vi "Serial Interface.vi"(1 "UART Inputs":T2={"Tx Data"=[0, 0, 0, 0, 0, 0, 0, 0, 0, 0], "Transmit"=FALSE, "Receive"=FALSE, "Byte Mode"=TRUE, "Set Baud Rate"=FALSE, "Baud Rate"=0} {"Baud Rate" format="%02x"; "Tx Data" format="%02x"}) -> (0 "UART Outputs":T1 {"Rx Data" format="%02x"})   [LabVIEW 2016]
uses:
  <vilib>/rvi/eio/common/nirviEmuTemplateMethod_errors.vi
  <vilib>/eio/EIONode/EIONode.xnode
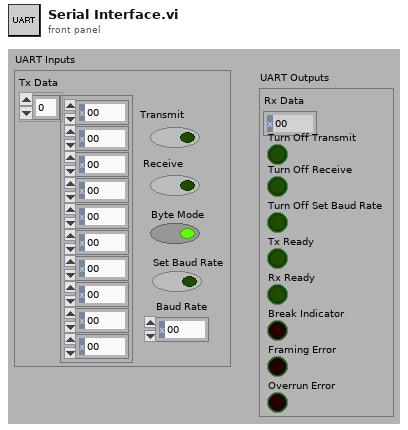
[diagram p1: front panel]
types:
  T1 = cluster{"Rx Data":u8, "Turn Off Transmit":bool, "Turn Off Receive":bool, "Turn Off Set Baud Rate":bool, "Tx Ready":bool, "Rx Ready":bool, "Break Indicator":bool, "Framing Error":bool, "Overrun Error":bool}
  T2 = cluster{"Tx Data":u8[], "Transmit":bool, "Receive":bool, "Byte Mode":bool, "Set Baud Rate":bool, "Baud Rate":u8}
  T3 = enum16{"Idle", "Assert Read", "Latch Data", "Done"}
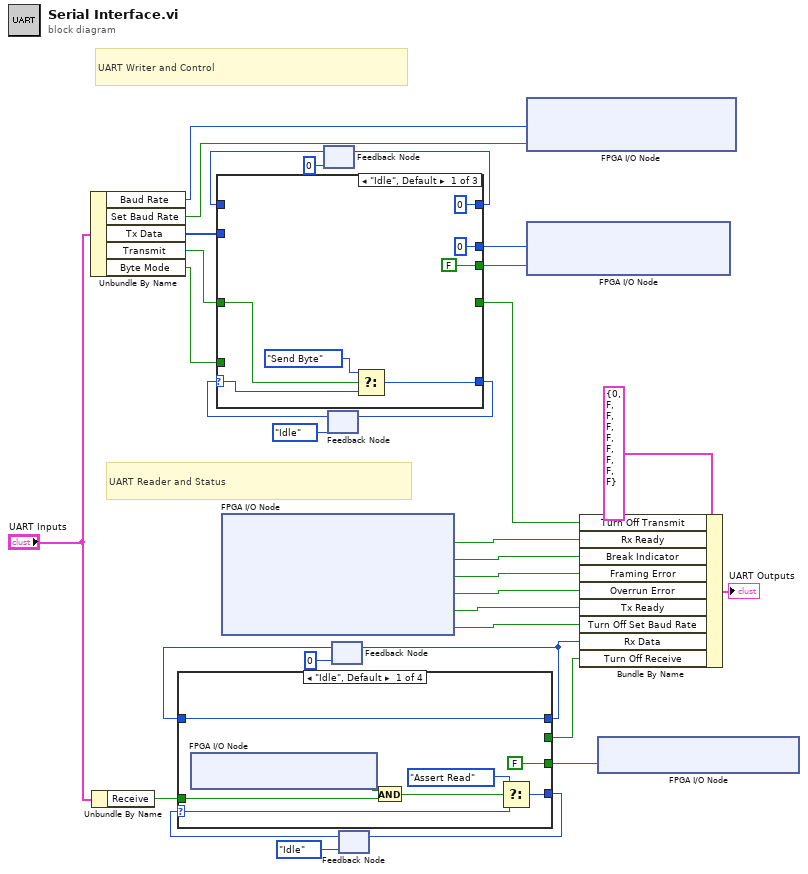
[diagram p0: block diagram]
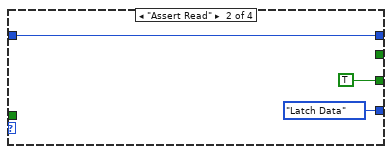
[diagram p2: hidden frame]
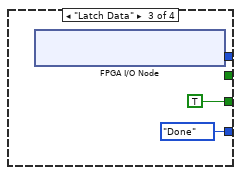
[diagram p3: hidden frame]
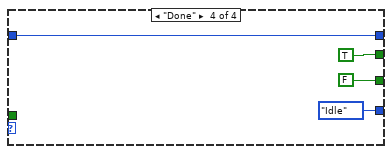
[diagram p4: hidden frame]
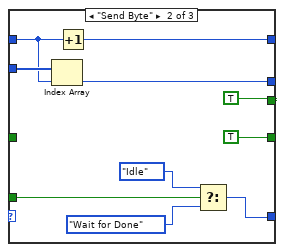
[diagram p5: hidden frame]
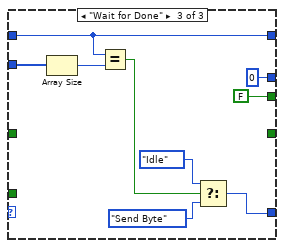
[diagram p6: hidden frame]
diagram:
  # "UART Writer and Control"
  # "UART Reader and Status"
  n1 = Unbundle By Name("UART Inputs") -> ("Baud Rate"=w6:u8, "Set Baud Rate"=w4:bool, "Tx Data"=w10:u8[], "Transmit"=w3:bool, "Byte Mode"=w9:bool)
  n2 = Unbundle By Name("UART Inputs") -> ("Receive"=w5:bool)
  n3 = xnode "FPGA I/O Node"() -> ("IO Module\\UART RX Ready"=w7:bool, "IO Module\\UART Break Indicator"=w18:bool, "IO Module\\UART Framing Error"=w17:bool, "IO Module\\UART RX Overrun Error"=w16:bool, "IO Module\\UART TX Ready"=w15:bool, "IO Module\\UART Set Baud Rate Ack"=w14:bool)  [unwired: 6 in, 6 out]
  n4 = feedback #1(u8 0) -> (w27:u8)
  n5 = feedback #2(enum16{"Idle", "Send Byte", "Wait for Done"}."Idle") -> (w29:enum16{"Idle", "Send Byte", "Wait for Done"})
  n6 = case shown="\"Idle\", Default" w29 {
    selector: w29 -> [w37 _ _]
    tunnel: w3 -> [w33 _ _]
    tunnel: [w39 w41 w54] -> w30
    tunnel: [FALSE TRUE FALSE] -> w25
    tunnel: w10 -> [_ w48 w56]
    tunnel: w27 -> [_ w47 w50]
    tunnel: [u8 0 w46 w50] -> w26
    tunnel: [u8 0 ("rUartDataIn") w45 u8 0 ("rUartDataIn")] -> w32
    tunnel: w9 -> [_ w43 _]
    tunnel: [_ TRUE _] -> w11
    frame "Idle", Default {
      n7 = Select(t=enum16{"Idle", "Send Byte", "Wait for Done"}."Send Byte", s=w33, f=w37) -> (s? t:f=w39:enum16{"Idle", "Send Byte", "Wait for Done"})
    }
    frame "Send Byte" {
      n8 = Index Array(array=w48, index=w47) -> (element=w45:u8)
      n9 = Increment(x=w47) -> (x+1=w46:u8)
      n10 = Select(t=enum16{"Idle", "Send Byte", "Wait for Done"}."Idle", s=w43, f=enum16{"Idle", "Send Byte", "Wait for Done"}."Wait for Done") -> (s? t:f=w41:enum16{"Idle", "Send Byte", "Wait for Done"})
    }
    frame "Wait for Done" {
      n11 = Array Size(array=w56) -> (size(s)=w51:i32)
      n12 = Equal?(x=w50, y=w51) -> (x = y?=w52:bool)
      n13 = Select(t=enum16{"Idle", "Send Byte", "Wait for Done"}."Idle", s=w52, f=enum16{"Idle", "Send Byte", "Wait for Done"}."Send Byte") -> (s? t:f=w54:enum16{"Idle", "Send Byte", "Wait for Done"})
    }
  }
  n14 = feedback-in #1(w26) -> ()
  n15 = feedback-in #2(w30) -> ()
  n16 = feedback #3(u8 0 ("IO Module\\rUartDataOut")) -> (w19:u8)
  n17 = feedback #4(T3."Idle") -> (w22:T3)
  n18 = case shown="\"Idle\", Default" w22 {
    selector: w22 -> [w65 _ _ _]
    tunnel: w5 -> [w60 _ _ _]
    tunnel: [w66 T3."Latch Data" ("t") T3."Done" ("t") T3."Idle" ("t")] -> w21
    tunnel: [FALSE TRUE TRUE FALSE] -> w24
    tunnel: [w62 w67 w70 w74] -> w12
    tunnel: w19 -> [w62 w67 _ w74]
    tunnel: [_ _ _ TRUE] -> w13
    frame "Idle", Default {
      n19 = xnode "FPGA I/O Node"() -> ("IO Module\\UART RX Ready"=w59:bool)  [unwired: 1 in, 1 out]
      n20 = And(x=w59, y=w60) -> (x .and. y?=w61:bool)
      n21 = Select(t=T3."Assert Read", s=w61, f=w65) -> (s? t:f=w66:T3)
    }
    frame "Assert Read" {
    }
    frame "Latch Data" {
      n22 = xnode "FPGA I/O Node"() -> ("IO Module\\UART Read Data"=w70:u8)  [unwired: 1 in, 1 out]
    }
    frame "Done" {
    }
  }
  n23 = feedback-in #3(w12) -> ()
  n24 = feedback-in #4(w21) -> ()
  n25 = xnode "FPGA I/O Node"("IO Module\\UART Baud Rate In"=w6, "IO Module\\UART Set Baud Rate"=w4) -> ()  [unwired: 2 in, 2 out]
  n26 = xnode "FPGA I/O Node"("IO Module\\UART Write Data"=w32, "IO Module\\UART Write Enable"=w25) -> ()  [unwired: 2 in, 2 out]
  n27 = Bundle By Name(cluster=T1 {"Rx Data"=0, "Turn Off Transmit"=FALSE, "Turn Off Receive"=FALSE, "Turn Off Set Baud Rate"=FALSE, "Tx Ready"=FALSE, "Rx Ready"=FALSE, "Break Indicator"=FALSE, "Framing Error"=FALSE, "Overrun Error"=FALSE} ("UART Outputs"), "Turn Off Transmit"=w11, "Rx Ready"=w7, "Break Indicator"=w18, "Framing Error"=w17, "Overrun Error"=w16, "Tx Ready"=w15, "Turn Off Set Baud Rate"=w14, "Rx Data"=w12, "Turn Off Receive"=w13) -> (→"UART Outputs":T1)
  n28 = xnode "FPGA I/O Node"("IO Module\\UART Read Enable"=w24) -> ()  [unwired: 1 in, 1 out]
